vi "DeleteWaveformsList.vi"(1 "Delete Waveform Options":u16(ring) items=["Waveform Name", "All (Only Imported Waveforms)"], 3 "error in (no error)":errorcluster, 4 "Delete Waveform from Waveform List (Name)":string, 5 "VISA resource name":refnum<visa-resource-name>) -> (0 "error out":errorcluster, 2 "VISA resource name out":refnum<visa-resource-name>)   [LabVIEW 2020, in "Active Technologies AWG3000.lvlib"]
uses:
  Active Technologies AWG3000.lvlib
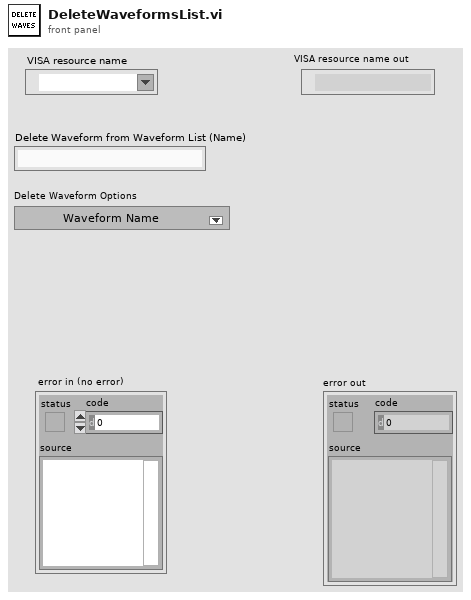
[diagram p1: front panel]
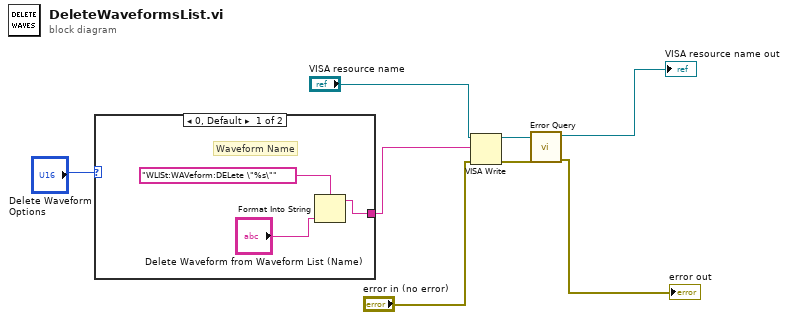
[diagram p0: block diagram]
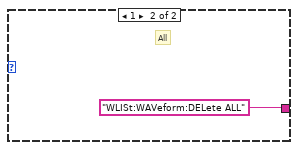
[diagram p2: hidden frame]
diagram:
  n1 = case shown="0, Default" "Delete Waveform Options" {
    tunnel: [w9 "WLISt:WAVeform:DELete ALL" ("write buffer")] -> w1
    frame 0, Default {
      # "Waveform Name"
      n2 = Format Into String(format string="WLISt:WAVeform:DELete \"%s\"" ("write buffer"), "Delete Waveform from Waveform List (Name)") -> (resulting string=w9:string)  [unwired: 2 in, 1 out]
    }
    frame 1 {
      # "All"
    }
  }
  n3 = VISA Write(VISA resource name="VISA resource name", write buffer=w1, error in (no error)="error in (no error)") -> (VISA resource name out=w6:refnum<visa-resource-name>, error out=w5:errorcluster)  [unwired: 1 out]
  n4 = call "Error Query.vi"("error in (no error)"=w5, "VISA resource name"=w6) -> ("error out"=→"error out":errorcluster, "VISA resource name out"=→"VISA resource name out":refnum<visa-resource-name>)  [unwired: 6 in, 2 out]
